vi "InitializePIDParams.vi"(0 "DAQ_QPT_Throlab in":refnum<class "DAQ_QPD_Throlab.lvclass">, 5 "PIDParams.Kp":dbl, 7 "PIDParams.Ki":dbl, 9 "PIDParams.Kd":dbl, 11 "error in (no error)":errorcluster) -> (4 "DAQ_QPT_Throlab out":refnum<class "DAQ_QPD_Throlab.lvclass">, 15 "error out":errorcluster)   [LabVIEW 2020, in "DAQ_QPD_Throlab.lvlib" / "DAQ_QPD_Throlab.lvclass"]
uses:
  DAQ_QPD_Throlab.lvclass
  DAQ_QPD_Throlab.lvclass/DAQ_QPD_Throlab.ctl
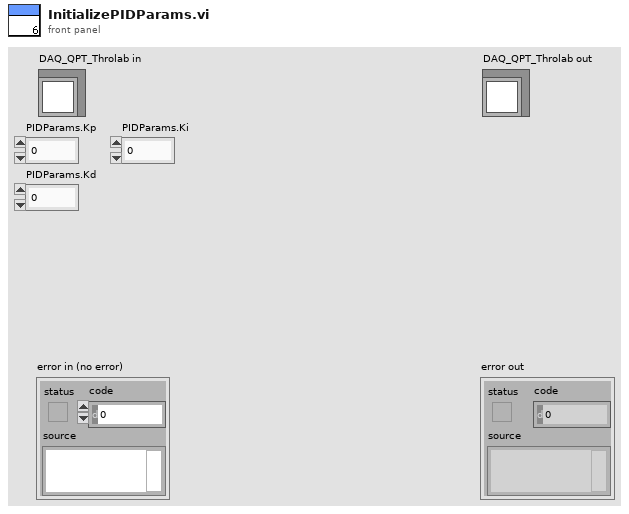
[diagram p1: front panel]
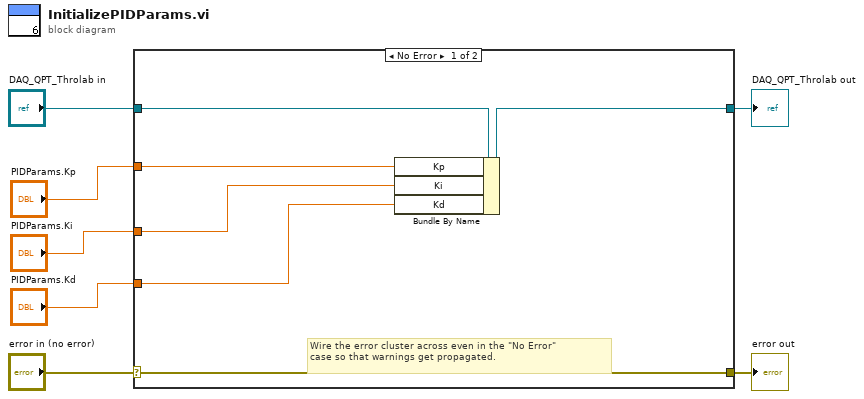
[diagram p0: block diagram]
diagram:
  n1 = case shown="No Error" "error in (no error)" {
    selector: "error in (no error)" -> [w12 w15]
    tunnel: [w12 w15] -> w6
    tunnel: [w11 w14] -> w4
    tunnel: "DAQ_QPT_Throlab in" -> [w13 w14]
    tunnel: "PIDParams.Kd" -> [w10 _]
    tunnel: "PIDParams.Ki" -> [w9 _]
    tunnel: "PIDParams.Kp" -> [w8 _]
    frame No Error {
      # "Wire the error cluster across even in the \"No Error\"\ncase so that warnings get propagated."
      n2 = Bundle By Name(cluster=w13, "Kp"=w8, "Ki"=w9, "Kd"=w10) -> (w11:refnum<class "DAQ_QPD_Throlab.lvclass">)
    }
    frame Error {
    }
  }
  "error out" <- w6
  "DAQ_QPT_Throlab out" <- w4
